vi "PingPong.IncReadAddr.vi"(8 "INC?":bool, 10 "Reset?":bool, 11 "rollover":u16) -> (0 "Output Valid":bool, 1 "roll over":bool, 3 "count":u16)   [LabVIEW 2014]
doc: "This counter counts from 0....Rollover and then returns to zero\ne.g., If rollover is 2, counter moves as 0,1,2,0,1,2.....\n\n<Latency> = 1 Tick from Reset"
panel:
  # "Copyright 2014 Vidrio Technologies\nScanImage 5 software is licensed under the Apache License, Version 2.0 (the \"License\"); you may not use any files contained\nwithin the ScanImage 5 release except in compliance with the License. You may obtain a copy of the License at\n http://www.apache.org/licenses/LICENSE-2.0\nUnless required by applicable law or agreed to in writing, software distributed under the License is distributed on an\n\"AS IS\" BASIS, WITHOUT WARRANTIES OR CONDITIONS OF ANY KIND, either express or implied. See the License for the\n specific language governing permissions and limitations under the License."
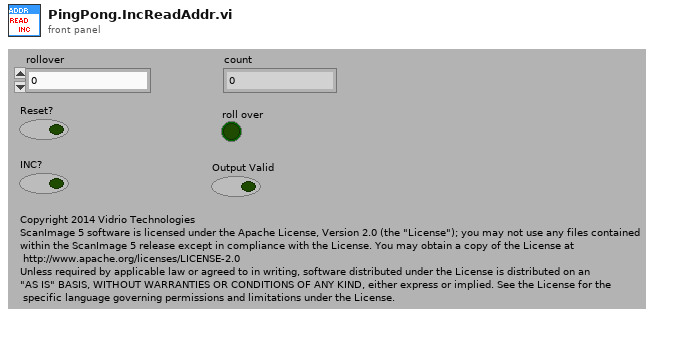
[diagram p1: front panel]
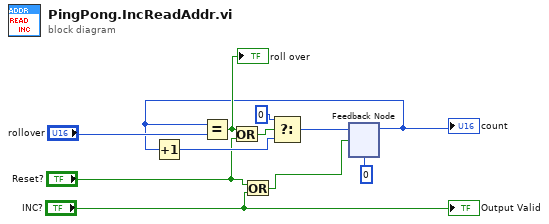
[diagram p0: block diagram]
diagram:
  n1 = Or(x="Reset?", y="INC?") -> (x .or. y?=w1:bool)
  n2 = feedback #1(u16 0) -> (w4:u16)
  "count" <- w4
  n3 = Increment(x=w4) -> (x+1=w6:u16)
  n4 = Equal?(x=w4, y="rollover") -> (x = y?=w9:bool)
  "roll over" <- w9
  n5 = Or(x=w9, y="Reset?") -> (x .or. y?=w8:bool)
  n6 = Select(t=u16 0, s=w8, f=w6) -> (s? t:f=w7:u16)
  n7 = feedback-in #1(w7, w1) -> ()
  "Output Valid" <- "INC?"
